vi "LOGIN.vi"() -> ()   [LabVIEW 2024]
uses:
  <vilib>/Utility/config.llb/NI_LVConfig.lvlib
  <vilib>/Utility/config.llb/Read Key (String).vi
panel:
  in  "USER NAME":string
  in  "PASSWORD":string
  in  "LOGIN":bool
  # "EOL TEST BENCH FOR THERMISTOR"
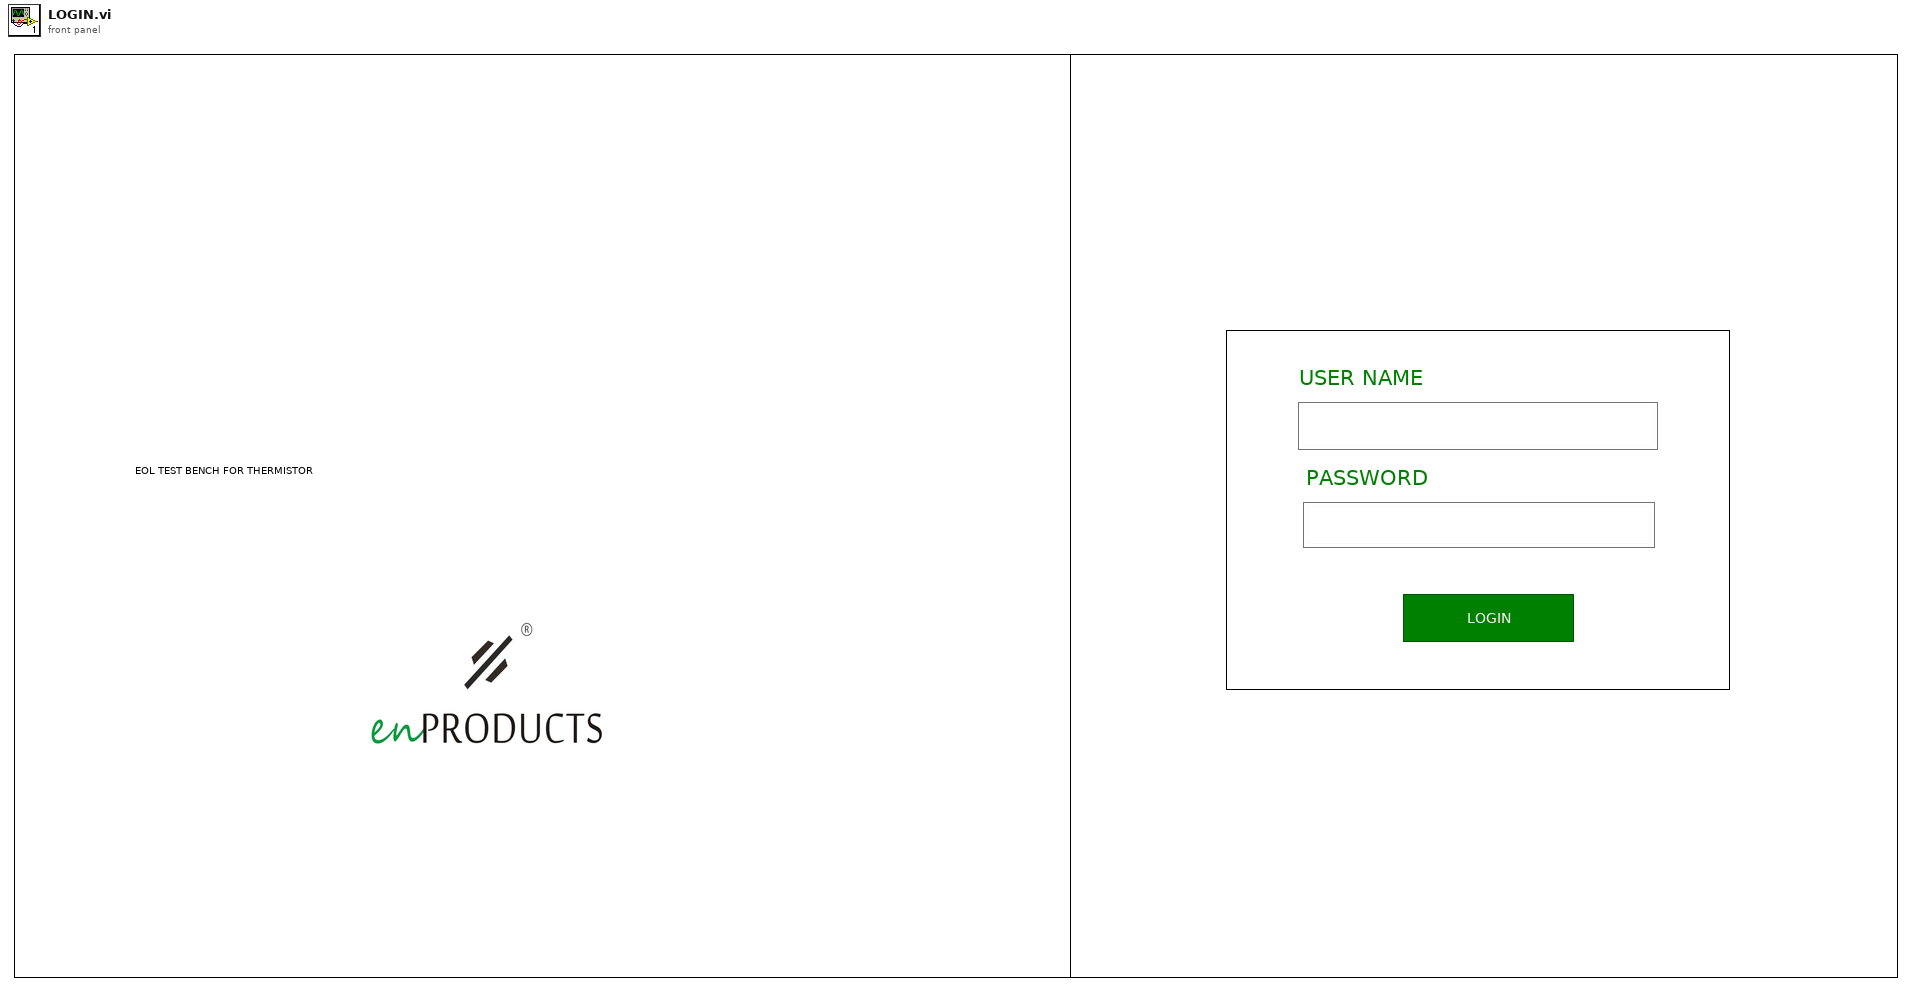
[diagram p1: front panel]
types:
  T1 = enum16{"TIME OUT", "INITIALIZE", "LOGIN", "PASSWORD CHECK", "PAGE NAVIGATION"}
  T2 = enum32{"Invalid", "Standard", "Closed", "Hidden", "Minimized", "Maximized"}
  T3 = typedef "NI_LVConfig.lvlib/Config Data RefNum.ctl" = refnum<k1>
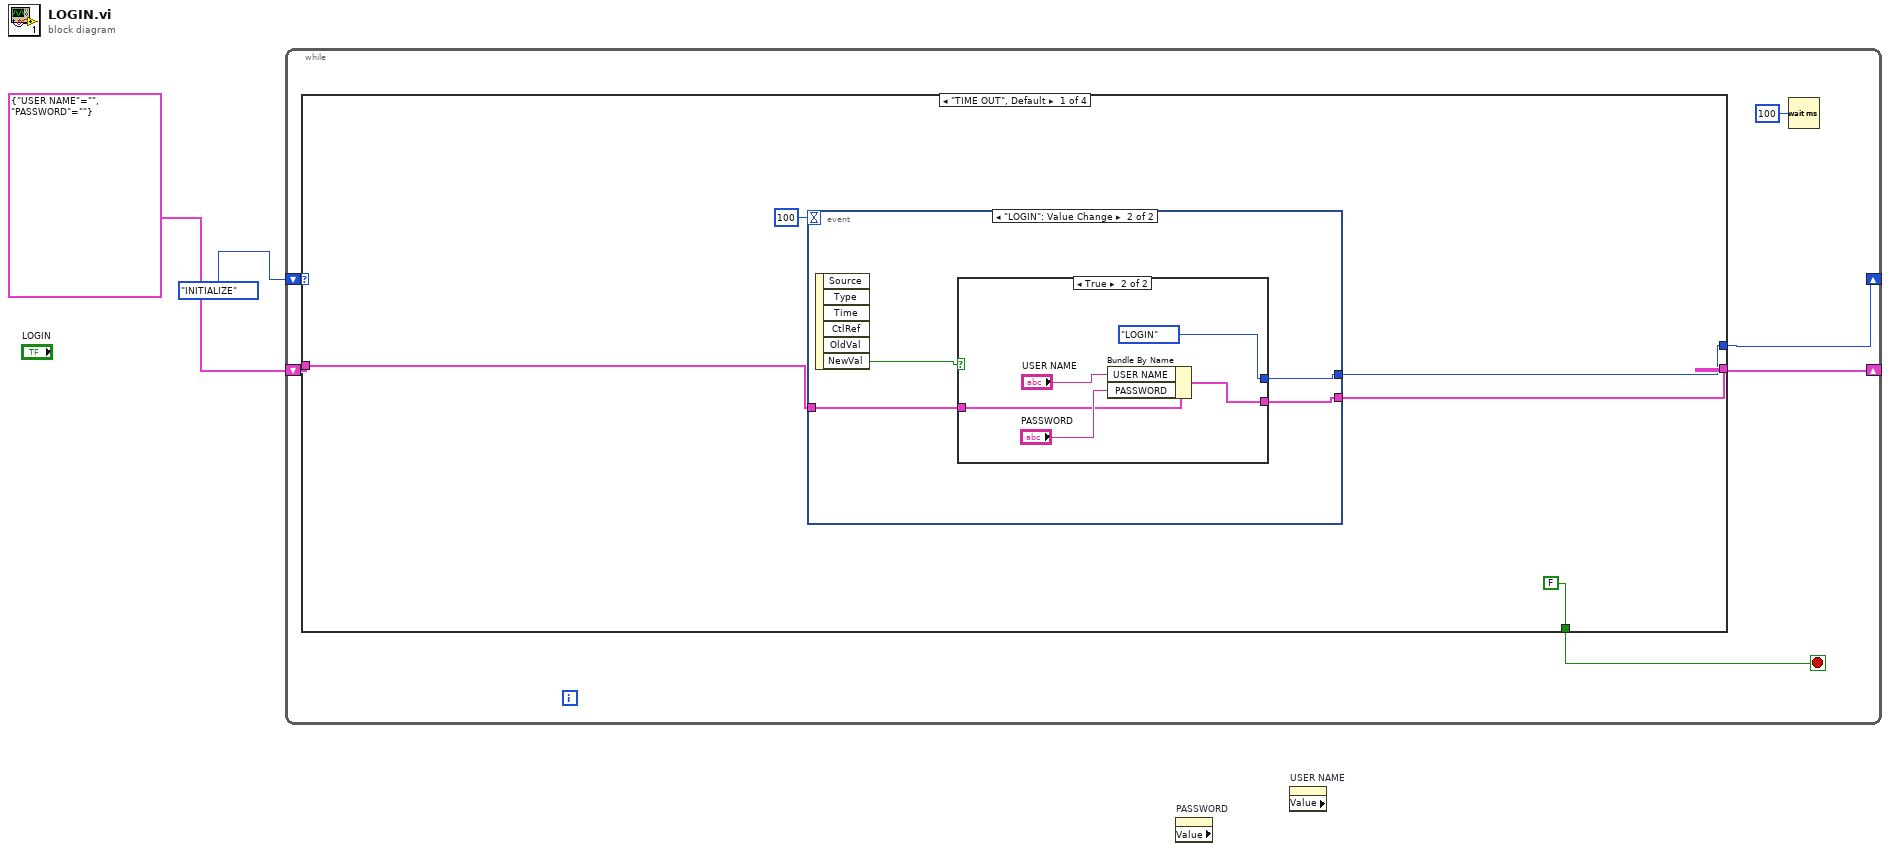
[diagram p0: block diagram]
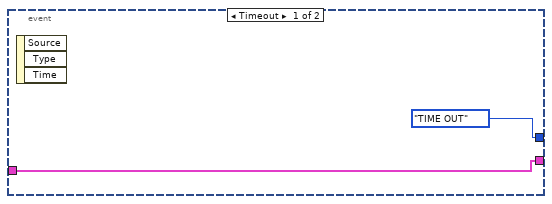
[diagram p2: hidden frame]
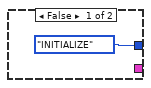
[diagram p3: hidden frame]
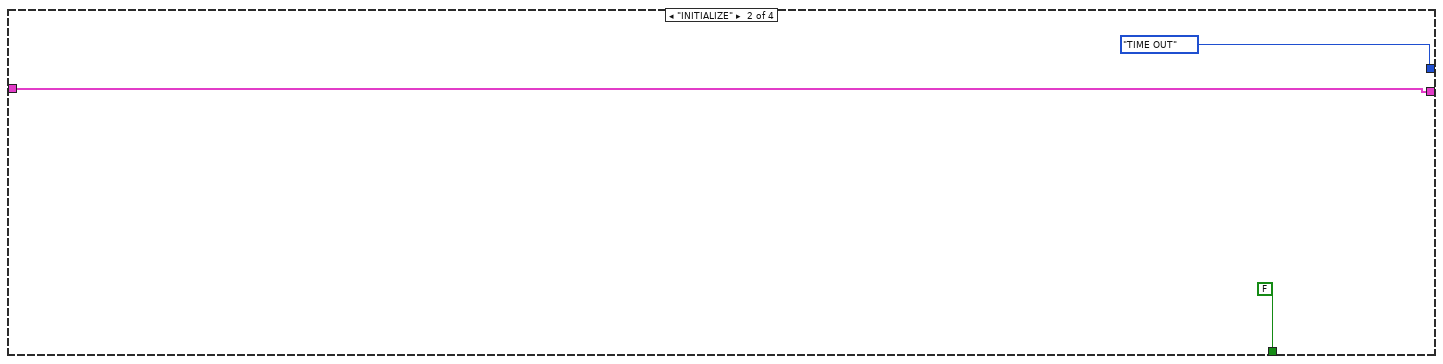
[diagram p4: hidden frame]
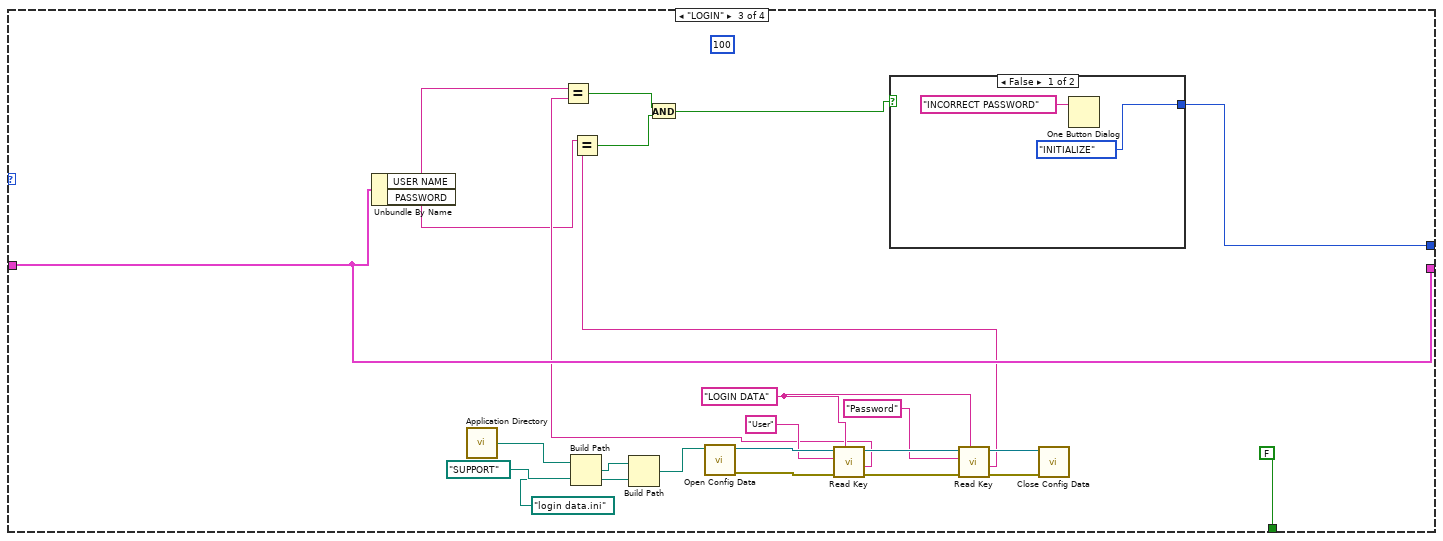
[diagram p5: hidden frame]
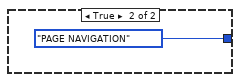
[diagram p6: hidden frame]
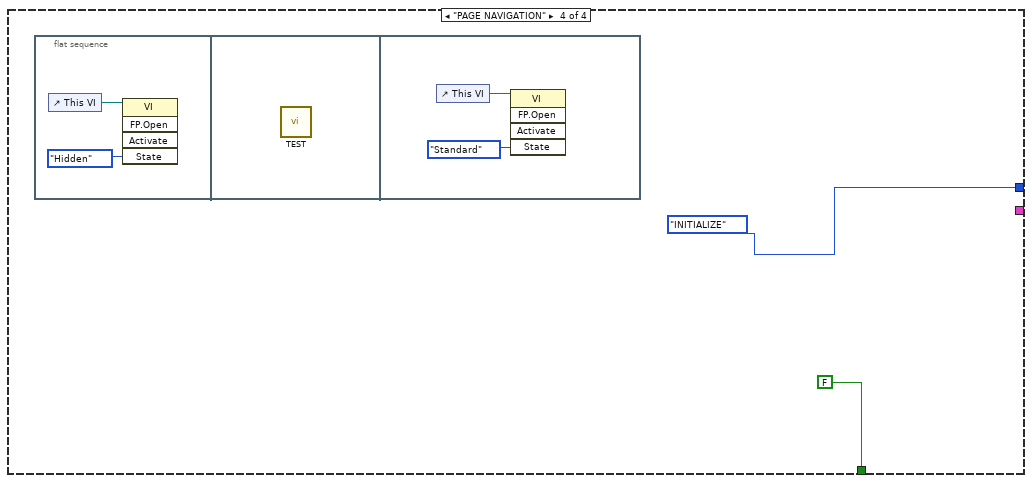
[diagram p7: hidden frame]
diagram:
  n1 = while {
    shift-right: [w7] -> _
    shift-left: T1."INITIALIZE" -> [w8]
    shift-right: [w5] -> _
    shift-left: cluster{"USER NAME":string, "PASSWORD":string} {"USER NAME"="", "PASSWORD"=""} -> [w6]
    stop <- w4 stop-if-true
    n2 = case shown="\"TIME OUT\", Default" w8 {
      tunnel: [w11 T1."TIME OUT" w39 T1."INITIALIZE"] -> w7
      tunnel: w6 -> [w12 w27 w43 _]
      tunnel: [w10 w27 w43 _] -> w5
      tunnel: [FALSE FALSE FALSE FALSE] -> w4
      frame "TIME OUT", Default {
        n3 = event shown="[1] \"LOGIN\": Value Change" {
          selector: _ -> [_ _]
          dyn-events: _ -> [_ _]
          timeout: 100 -> [_ _]
          tunnel: [T1."TIME OUT" w17] -> w11
          tunnel: w12 -> [w14 w18]
          tunnel: [w14 w19] -> w10
          event Timeout {
            n4 = event-data() -> ()  [unwired: 1 in, 3 out]
          }
          event "LOGIN": Value Change {
            n5 = event-data() -> ("NewVal"=w16:bool)  [unwired: 1 in, 5 out]
            n6 = case shown="True" w16 {
              tunnel: [T1."INITIALIZE" T1."LOGIN"] -> w17
              tunnel: [_ w23] -> w19
              tunnel: w18 -> [_ w21]
              frame False {
              }
              frame True {
                n7 = Bundle By Name(cluster=w21, "USER NAME"="USER NAME", "PASSWORD"="PASSWORD") -> (w23:cluster{"USER NAME":string, "PASSWORD":string})
              }
            }
          }
        }
      }
      frame "INITIALIZE" {
      }
      frame "LOGIN" {
        (unwired) 100
        w46 = "LOGIN DATA" ("section")
        n8 = Unbundle By Name(w43) -> ("USER NAME"=w42:string, "PASSWORD"=w40:string)
        n9 = call <vilib>:"Application Directory.vi"() -> ("Application Directory"=w33:path)
        n10 = Build Path(base path=w33, name or relative path=path "SUPPORT") -> (appended path=w31:path)
        n11 = Build Path(base path=w31, name or relative path=path "login data.ini") -> (appended path=w29:path)
        n12 = call <vilib>:"Open Config Data.vi"("configuration file path"=w29) -> ("error out"=w49:errorcluster, "refnum"=w52:T3)  [unwired: 8 in, 1 out]
        n13 = call-poly <vilib>:"Read Key.vi"("section"=w46, "error in (no error)"=w49, "key"="User", "refnum"=w52) -> ("error out"=w48:errorcluster, "value"=w41:string, "refnum out"=w51:T3)  [unwired: 4 in, 1 out]
        n14 = Equal?(x=w42, y=w41) -> (x = y?=w37:bool)
        n15 = call-poly <vilib>:"Read Key.vi"("section"=w46, "error in (no error)"=w48, "key"="Password", "refnum"=w51) -> ("error out"=w47:errorcluster, "value"=w38:string, "refnum out"=w50:T3)  [unwired: 4 in, 1 out]
        n16 = Equal?(x=w40, y=w38) -> (x = y?=w36:bool)
        n17 = And(x=w37, y=w36) -> (x .and. y?=w35:bool)
        n18 = case shown="False" w35 {
          tunnel: [T1."INITIALIZE" T1."PAGE NAVIGATION"] -> w39
          frame False {
            n19 = One Button Dialog(message="INCORRECT PASSWORD") -> ()  [unwired: 1 in, 1 out]
          }
          frame True {
          }
        }
        n20 = call <vilib>:"Close Config Data.vi"("error in (no error)"=w47, "refnum"=w50) -> ()  [unwired: 8 in, 2 out]
      }
      frame "PAGE NAVIGATION" {
        n21 = flat-sequence {
          frame #0 {
            n22 = control-ref of="This VI"() -> (w59:refnum<vi>)
            n23 = invoke class="VI" method="FP.Open"(reference=w59, "State"=T2."Hidden") -> ()  [unwired: 3 in, 5 out]
          }
          frame #1 {
            n24 = call "TEST.vi"() -> ()  [unwired: 12 in]
          }
          frame #2 {
            n25 = control-ref of="This VI"() -> (w61:refnum<vi>)
            n26 = invoke class="VI" method="FP.Open"(reference=w61, "State"=T2."Standard") -> ()  [unwired: 3 in, 5 out]
          }
        }
      }
    }
    n27 = Wait (ms)(milliseconds to wait=u32 100) -> ()  [unwired: 1 out]
  }
  n28 = property on="PASSWORD" class="Str" props=["Value"]() -> ()  [unwired: 2 in, 3 out]
  n29 = property on="USER NAME" class="Str" props=["Value"]() -> ()  [unwired: 2 in, 3 out]
